vi "Release Semaphore_71.vi"(4 "error in (no error)":errorcluster, 7 "semaphore":T1) -> (0 "error out":errorcluster, 3 "semaphore out":T1)   [LabVIEW 2020]
doc: "Releases access to a semaphore."
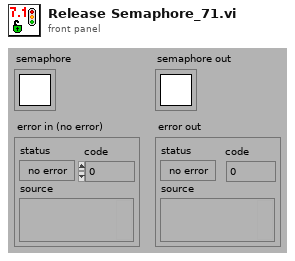
[diagram p1: front panel]
types:
  T1 = typedef "Semaphore RefNum" = refnum<k1>
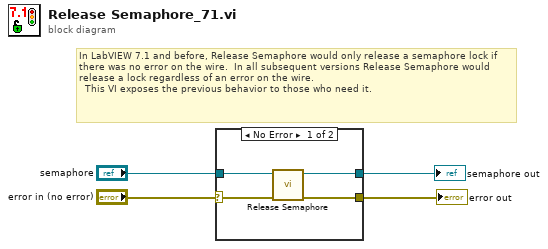
[diagram p0: block diagram]
diagram:
  # "In LabVIEW 7.1 and before, Release Semaphore would only release a semaphore lock if there was no error on the wire.  In all subsequent versions Release Semaphore would release a lock regardless of an error on the wire.\n  This VI exposes the previous behavior to those who need it."
  n1 = case shown="No Error" "error in (no error)" {
    selector: "error in (no error)" -> [w6 w9]
    tunnel: [w5 w9] -> w3
    tunnel: [w7 w10] -> w2
    tunnel: "semaphore" -> [w8 w10]
    frame No Error {
      n2 = call "Release Semaphore.vi"("error in (no error)"=w6, "semaphore"=w8) -> ("error out"=w5:errorcluster, "semaphore out"=w7:T1)  [unwired: 4 out]
    }
    frame Error {
    }
  }
  "semaphore out" <- w2
  "error out" <- w3
